vi "Sensor_Initialization.vi"   [LabVIEW 2018]
uses:
  <vilib>/Rock Robotics/SystemInterfaces/DIO/FPGA_DIOChannel.ctl
  <vilib>/Rock Robotics/SystemInterfaces/AI/FPGA_AIChannel.ctl
  <vilib>/Rock Robotics/WPI/Switch/WPI_SwitchOpenLimit.vi
  Global_Variables/Drive_Globals.vi
  Global_Variables/Intake_Joint_Globals.vi
  Global_Variables/Elevator_Globals.vi
  Global_Variables/Climb_Globals.vi
types:
  T1 = typedef "FPGA_AIChannel.ctl" = enum8{"AI 0", "AI 1", "AI 2", "AI 3", "AI MXP 0", "AI MXP 1", "AI MXP 2", "AI MXP 3", "Invalid"}
  T2 = typedef "FPGA_DIOChannel.ctl" = enum8{"DIO 0", "DIO 1", "DIO 2", "DIO 3", "DIO 4", "DIO 5", "DIO 6", "DIO 7", "DIO 8", "DIO 9", "DIO MXP 0", "DIO MXP 1", "DIO MXP 2", "DIO MXP 3", "DIO MXP 4", "DIO MXP 5", "DIO MXP 6", "DIO MXP 7", "DIO MXP 8", "DIO MXP 9", "DIO MXP 10", "DIO MXP 11", "DIO MXP 12", "DIO MXP 13", "DIO MXP 14", "DIO MXP 15", "SPI Port CS1", "SPI Port CS2", "SPI Port CS3", "SPI Port MISO", "SPI Port MOSI", "Invalid"}
  T3 = typedef "WPI_SwitchDevRef.ctl" = cluster{"DevStatus":errorcluster, "DIO Channel":T2, "CntIndex":T4, "Normally Closed":bool}
  T4 = typedef "FPGA_CounterCtrSystemIndex.ctl" = enum8{"Ctr 0", "Ctr 1", "Ctr 2", "Ctr 3", "Ctr 4", "Ctr 5", "Ctr 6", "Ctr 7", "Invalid"}
  T5 = typedef "WPI_AnalogChannelDevRef.ctl" = cluster{"DevStatus":errorcluster, "Analog Channel":T1}
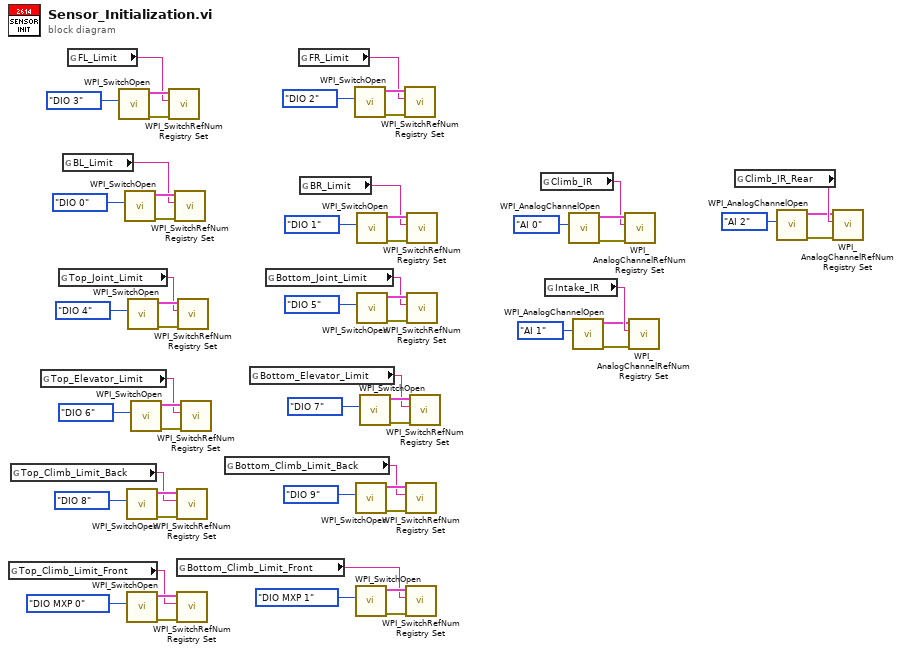
[diagram p0: block diagram]
diagram:
  n1 = global read "Elevator_Globals.vi" "Top_Climb_Limit_Front"() -> (w14:string)
  n2 = global read "Climb_Globals.vi" "Top_Climb_Limit_Back"() -> (w10:string)
  n3 = global read "Elevator_Globals.vi" "Top_Elevator_Limit"() -> (w12:string)
  n4 = global read "Intake_Joint_Globals.vi" "Top_Joint_Limit"() -> (w16:string)
  n5 = global read "Drive_Globals.vi" "BL_Limit"() -> (w47:string)
  n6 = global read "Drive_Globals.vi" "FL_Limit"() -> (w48:string)
  n7 = call-poly <vilib>:"WPI_SwitchOpen.vi"("DIO Channel"=FPGA_DIOChannel."DIO 3") -> ("error out"=w59:errorcluster, "SwitchDevRef"=w60:T3)  [unwired: 9 in]
  n8 = call-poly <vilib>:"WPI_SwitchOpen.vi"("DIO Channel"=FPGA_DIOChannel."DIO 0") -> ("error out"=w53:errorcluster, "SwitchDevRef"=w54:T3)  [unwired: 9 in]
  n9 = call-poly <vilib>:"WPI_SwitchOpen.vi"("DIO Channel"=FPGA_DIOChannel."DIO 8") -> ("error out"=w40:errorcluster, "SwitchDevRef"=w39:T3)  [unwired: 9 in]
  n10 = call-poly <vilib>:"WPI_SwitchOpen.vi"("DIO Channel"=FPGA_DIOChannel."DIO MXP 0") -> ("error out"=w37:errorcluster, "SwitchDevRef"=w38:T3)  [unwired: 9 in]
  n11 = call-poly <vilib>:"WPI_SwitchOpen.vi"("DIO Channel"=FPGA_DIOChannel."DIO 4") -> ("error out"=w22:errorcluster, "SwitchDevRef"=w21:T3)  [unwired: 9 in]
  n12 = call-poly <vilib>:"WPI_SwitchOpen.vi"("DIO Channel"=FPGA_DIOChannel."DIO 6") -> ("error out"=w31:errorcluster, "SwitchDevRef"=w32:T3)  [unwired: 9 in]
  n13 = call <vilib>:"WPI_SwitchRefNum Registry Set.vi"("error in (no error)"=w59, "refnum name"=w48, "SwitchDevRef"=w60) -> ()  [unwired: 7 in, 2 out]
  n14 = call <vilib>:"WPI_SwitchRefNum Registry Set.vi"("error in (no error)"=w53, "refnum name"=w47, "SwitchDevRef"=w54) -> ()  [unwired: 7 in, 2 out]
  n15 = call <vilib>:"WPI_SwitchRefNum Registry Set.vi"("error in (no error)"=w40, "refnum name"=w10, "SwitchDevRef"=w39) -> ()  [unwired: 7 in, 2 out]
  n16 = global read "Elevator_Globals.vi" "Bottom_Climb_Limit_Front"() -> (w15:string)
  n17 = call <vilib>:"WPI_SwitchRefNum Registry Set.vi"("error in (no error)"=w37, "refnum name"=w14, "SwitchDevRef"=w38) -> ()  [unwired: 7 in, 2 out]
  n18 = call <vilib>:"WPI_SwitchRefNum Registry Set.vi"("error in (no error)"=w22, "refnum name"=w16, "SwitchDevRef"=w21) -> ()  [unwired: 7 in, 2 out]
  n19 = call <vilib>:"WPI_SwitchRefNum Registry Set.vi"("error in (no error)"=w31, "refnum name"=w12, "SwitchDevRef"=w32) -> ()  [unwired: 7 in, 2 out]
  n20 = global read "Climb_Globals.vi" "Bottom_Climb_Limit_Back"() -> (w11:string)
  n21 = global read "Elevator_Globals.vi" "Bottom_Elevator_Limit"() -> (w13:string)
  n22 = global read "Intake_Joint_Globals.vi" "Bottom_Joint_Limit"() -> (w17:string)
  n23 = global read "Drive_Globals.vi" "FR_Limit"() -> (w45:string)
  n24 = global read "Drive_Globals.vi" "BR_Limit"() -> (w46:string)
  n25 = call-poly <vilib>:"WPI_SwitchOpen.vi"("DIO Channel"=FPGA_DIOChannel."DIO 2") -> ("error out"=w56:errorcluster, "SwitchDevRef"=w55:T3)  [unwired: 9 in]
  n26 = call-poly <vilib>:"WPI_SwitchOpen.vi"("DIO Channel"=FPGA_DIOChannel."DIO 9") -> ("error out"=w43:errorcluster, "SwitchDevRef"=w44:T3)  [unwired: 9 in]
  n27 = call-poly <vilib>:"WPI_SwitchOpen.vi"("DIO Channel"=FPGA_DIOChannel."DIO MXP 1") -> ("error out"=w34:errorcluster, "SwitchDevRef"=w33:T3)  [unwired: 9 in]
  n28 = call-poly <vilib>:"WPI_SwitchOpen.vi"("DIO Channel"=FPGA_DIOChannel."DIO 1") -> ("error out"=w50:errorcluster, "SwitchDevRef"=w49:T3)  [unwired: 9 in]
  n29 = call-poly <vilib>:"WPI_SwitchOpen.vi"("DIO Channel"=FPGA_DIOChannel."DIO 5") -> ("error out"=w25:errorcluster, "SwitchDevRef"=w26:T3)  [unwired: 9 in]
  n30 = call-poly <vilib>:"WPI_SwitchOpen.vi"("DIO Channel"=FPGA_DIOChannel."DIO 7") -> ("error out"=w28:errorcluster, "SwitchDevRef"=w27:T3)  [unwired: 9 in]
  n31 = call <vilib>:"WPI_SwitchRefNum Registry Set.vi"("error in (no error)"=w56, "refnum name"=w45, "SwitchDevRef"=w55) -> ()  [unwired: 7 in, 2 out]
  n32 = call <vilib>:"WPI_SwitchRefNum Registry Set.vi"("error in (no error)"=w43, "refnum name"=w11, "SwitchDevRef"=w44) -> ()  [unwired: 7 in, 2 out]
  n33 = call <vilib>:"WPI_SwitchRefNum Registry Set.vi"("error in (no error)"=w34, "refnum name"=w15, "SwitchDevRef"=w33) -> ()  [unwired: 7 in, 2 out]
  n34 = call <vilib>:"WPI_SwitchRefNum Registry Set.vi"("error in (no error)"=w50, "refnum name"=w46, "SwitchDevRef"=w49) -> ()  [unwired: 7 in, 2 out]
  n35 = call <vilib>:"WPI_SwitchRefNum Registry Set.vi"("error in (no error)"=w25, "refnum name"=w17, "SwitchDevRef"=w26) -> ()  [unwired: 7 in, 2 out]
  n36 = call <vilib>:"WPI_SwitchRefNum Registry Set.vi"("error in (no error)"=w28, "refnum name"=w13, "SwitchDevRef"=w27) -> ()  [unwired: 7 in, 2 out]
  n37 = global read "Climb_Globals.vi" "Climb_IR"() -> (w9:string)
  n38 = global read "Climb_Globals.vi" "Intake_IR"() -> (w8:string)
  n39 = call <vilib>:"WPI_AnalogChannelOpen.vi"("Analog Channel"=FPGA_AIChannel."AI 0") -> ("error out"=w20:errorcluster, "AIDeviceRef"=w19:T5)  [unwired: 9 in]
  n40 = call <vilib>:"WPI_AnalogChannelOpen.vi"("Analog Channel"=FPGA_AIChannel."AI 1") -> ("error out"=w5:errorcluster, "AIDeviceRef"=w6:T5)  [unwired: 9 in]
  n41 = call <vilib>:"WPI_AnalogChannelRefNum Registry Set.vi"("error in (no error)"=w20, "refnum name"=w9, "AIDeviceRef"=w19) -> ()  [unwired: 7 in, 2 out]
  n42 = call <vilib>:"WPI_AnalogChannelRefNum Registry Set.vi"("error in (no error)"=w5, "refnum name"=w8, "AIDeviceRef"=w6) -> ()  [unwired: 7 in, 2 out]
  n43 = global read "Climb_Globals.vi" "Climb_IR_Rear"() -> (w4:string)
  n44 = call <vilib>:"WPI_AnalogChannelOpen.vi"("Analog Channel"=FPGA_AIChannel."AI 2") -> ("error out"=w1:errorcluster, "AIDeviceRef"=w2:T5)  [unwired: 9 in]
  n45 = call <vilib>:"WPI_AnalogChannelRefNum Registry Set.vi"("error in (no error)"=w1, "refnum name"=w4, "AIDeviceRef"=w2) -> ()  [unwired: 7 in, 2 out]
